vi "event.create.vi"(7 "Time Stamp (now)":timestamp format="%<%x %.3X>T", 8 "error in (no error)":errorcluster, 9 "Type":enum16{"INFO", "FLAG", "ERROR", "SUCCESS"}(ring), 10 "Name":string, 11 "Run in":refnum<class "Run.lvclass">) -> (0 "error out":errorcluster, 2 "event":refnum<class "event.lvclass">, 3 "Run out":refnum<class "Run.lvclass">)   [LabVIEW 2020, in "Run.lvclass"]
uses:
  Run.lvclass
  event/event.lvclass
  Run.lvclass/Run.ctl
  client.get.vi
  assets.get.vi
  assets.get.vi/fc990382-c15b-405e-8523-435b97eca7cf.vi
  assets.get.vi/fc990382-c15b-405e-8523-435b97eca7cf.vi/32c3acc2-0975-485a-8283-62feb0f3dc4f.vi
  run_properties.get.vi
  update.cache.vi
  <vilib>/JDP Science/JSONtext/JSON type.vi
  <vilib>/JDP Science/JSONtext/JSON text to Variant.vi
  Nominal Client/asset.get[].vi
  Nominal Client/Nominal Client.lvclass
  <vilib>/JDP Science/JSONtext/LVClass Serializer/JSONtext LVClass Serializer.lvclass
  asset/asset.lvclass
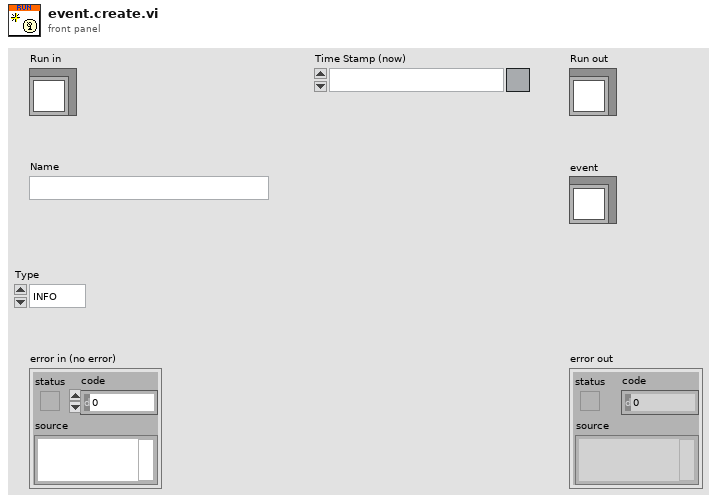
[diagram p1: front panel]
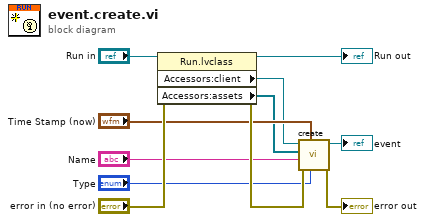
[diagram p0: block diagram]
diagram:
  n1 = property class="Run.lvclass"(reference="Run in", error in="error in (no error)") -> (reference out=→"Run out":refnum<class "Run.lvclass">, error out=w7:errorcluster, "Accessors:client"=w2:refnum<class "Nominal Client.lvclass">, "Accessors:assets"=w1:refnum<class "asset.lvclass">[])
  n2 = call "create.vi"("Type"="Type", "Time Stamp (now)"="Time Stamp (now)", "error in"=w7, "Name"="Name", "assets"=w1, "Nominal Client in"=w2) -> ("error out"=→"error out":errorcluster, "event"=→"event":refnum<class "event.lvclass">)  [unwired: 4 in]
